vi "Identify Pulse and Noise.vi"(8 "error in":errorcluster, 11 "Waveform In":waveform(dbl)) -> (0 "error out":errorcluster, 1 "Signal Waveform Out":waveform(dbl), 2 "Detected Frequency (Hz)":dbl, 3 "Noise Waveform Out":waveform(dbl), 4 "Pulse Start Time (ms)":dbl)   [LabVIEW 2020]
doc: "Seperates the noise from the signal, by spliting the data at the first peak."
uses:
  <vilib>/measure/mascope.llb/Transition Measurements 1 chan.vi
  <vilib>/Waveform/WDTOps.llb/WDT Get Waveform Subset DBL.vi
  <vilib>/measure/matone.llb/Extract Single Tone Information 1 Chan.vi
  <vilib>/measure/NI_MAPro.lvlib
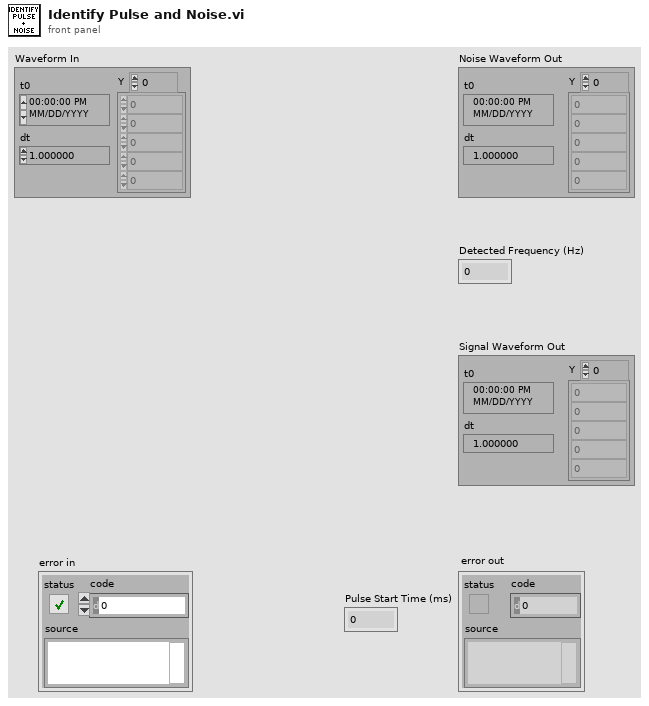
[diagram p1: front panel]
types:
  T1 = cluster{"start time":dbl, "end time":dbl, "ref levels":cluster{"high ref level":dbl, "mid ref level":dbl, "low ref level":dbl, "ref units":u16}}
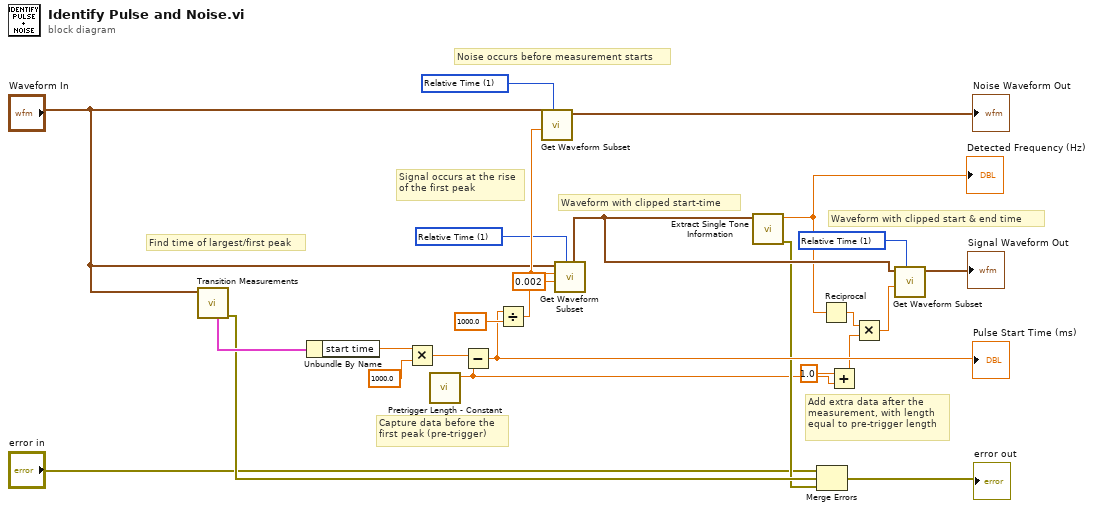
[diagram p0: block diagram]
diagram:
  w23 = u16 1 items=["Samples", "Relative Time"] ("start/duration format")
  w12 = u16 1 items=["Samples", "Relative Time"] ("start/duration format")
  w11 = u16 1 items=["Samples", "Relative Time"] ("start/duration format")
  # "Waveform with clipped start & end time"
  # "Waveform with clipped start-time"
  # "Find time of largest/first peak"
  # "Signal occurs at the rise\nof the first peak"
  # "Noise occurs before measurement starts"
  # "Capture data before the \nfirst peak (pre-trigger)"
  # "Add extra data after the\nmeasurement, with length\nequal to pre-trigger length"
  n1 = call-poly <vilib>:"Transition Measurements.vi"("signal in"="Waveform In") -> ("error out"=w7:errorcluster, "measurement info"=w8:T1)  [unwired: 5 in, 4 out]
  n2 = Unbundle By Name(w8) -> ("start time"=w13:dbl)
  n3 = Multiply(x=w13, y=1000.0) -> (x*y=w10:dbl)
  n4 = call "Pretrigger Length - Constant.vi"() -> ("Pretrigger length (fraction signal length)"=w3:dbl)  [unwired: 11 in]
  n5 = Subtract(x=w10, y=w3) -> (x-y=w16:dbl)
  "Pulse Start Time (ms)" <- w16
  n6 = Divide(x=w16, y=1000.0) -> (x/y=w18:dbl)
  n7 = call-poly <vilib>:"Get Waveform Subset.vi"("start/duration format"=w12, "duration"=w18, "waveform in"="Waveform In") -> ("waveform out"=→"Noise Waveform Out":waveform(dbl))  [unwired: 3 in, 3 out]
  n8 = call-poly <vilib>:"Get Waveform Subset.vi"("start/duration format"=w11, "duration"=0.002, "start samples/time"=w18, "waveform in"="Waveform In") -> ("waveform out"=w21:waveform(dbl))  [unwired: 2 in, 3 out]
  n9 = call-poly <vilib>:"Extract Single Tone Information.vi"("time signal in"=w21) -> ("error out"=w6:errorcluster, "detected frequency"=w20:dbl)  [unwired: 5 in, 4 out]
  "Detected Frequency (Hz)" <- w20
  n10 = Merge Errors("error in", w7, w6) -> (→"error out":errorcluster)
  n11 = Reciprocal(x=w20) -> (1/x=w24:dbl)
  n12 = Add(x=1.0, y=w3) -> (x+y=w1:dbl)
  n13 = Multiply(x=w24, y=w1) -> (x*y=w25:dbl)
  n14 = call-poly <vilib>:"Get Waveform Subset.vi"("start/duration format"=w23, "duration"=w25, "waveform in"=w21) -> ("waveform out"=→"Signal Waveform Out":waveform(dbl))  [unwired: 3 in, 3 out]
